vi "GetIOPinEnab.vi"(8 "错误输入（无错误）":errorcluster) -> (0 "错误输出":errorcluster, 3 "返回值":u8)   [LabVIEW 2014]
uses:
  X86Dll/ZXUTConfigMgr.dll
panel:
  in  "端口类型":i32
  in  "编码器序号":i32
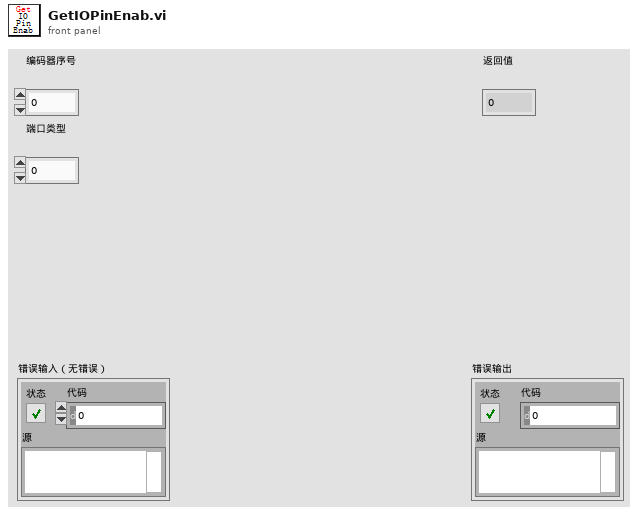
[diagram p1: front panel]
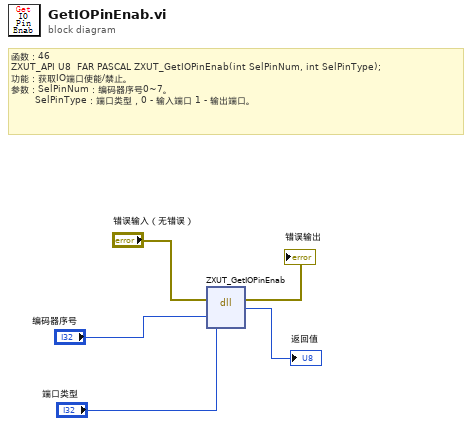
[diagram p0: block diagram]
diagram:
  # "函数：46\nZXUT_API U8\t\tFAR PASCAL ZXUT_GetIOPinEnab(int SelPinNum, int SelPinType);\n功能：获取IO端口使能/禁止。\n参数：SelPinNum：编码器序号0~7。\n        SelPinType：端口类型，0 - 输入端口 1 - 输出端口。"
  n1 = dll-call lib="D:/Software/Utrasonic on-line monitoring/X86Dll/ZXUTConfigMgr.dll" fn="ZXUT_GetIOPinEnab"(error in="错误输入（无错误）", "SelPinNum"="编码器序号", "SelPinType"="端口类型") -> (error out=→"错误输出":errorcluster, "返回值"=→"返回值":u8)  [unwired: 4 in, 1 out]
